vi "LED logic.vi"(11 "Blinks per cycle":i32) -> (3 "Boolean":bool)   [LabVIEW 2013, in "LED runtime.lvclass"]
uses:
  LED runtime.lvclass
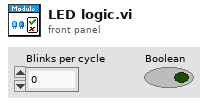
[diagram p1: front panel]
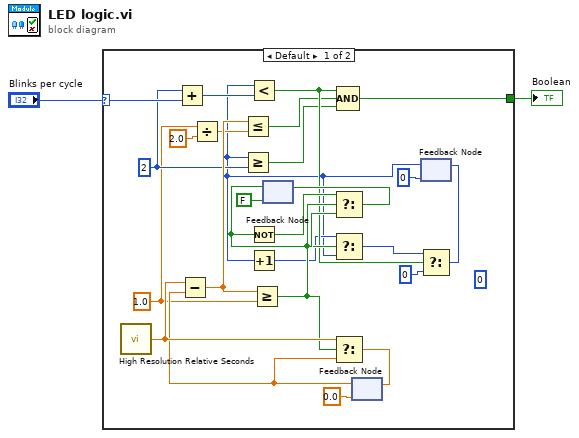
[diagram p0: block diagram]
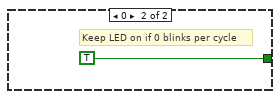
[diagram p2: hidden frame]
diagram:
  n1 = case shown="Default" "Blinks per cycle" {
    selector: "Blinks per cycle" -> [w9 _]
    tunnel: [w12 TRUE] -> w1
    frame Default {
      w3 = 1.0
      (unwired) 0 ("f")
      w7 = 2 ("x")
      n2 = call <vilib>:"High Resolution Relative Seconds.vi"() -> ("relative seconds"=w23:dbl)
      n3 = Add(x=w7, y=w9) -> (x+y=w8:i32)
      n4 = Divide(x=w3, y=2.0) -> (x/y=w13:dbl)
      n5 = feedback #1(FALSE) -> (w24:bool)
      n6 = Not(x=w24) -> (.not. x?=w26:bool)
      n7 = feedback #2(0.0) -> (w22:dbl)
      n8 = Subtract(x=w23, y=w22) -> (x-y=w15:dbl)
      n9 = Less Or Equal?(x=w15, y=w13) -> (x <= y?=w10:bool)
      n10 = Greater Or Equal?(x=w15, y=w3) -> (x >= y?=w17:bool)
      n11 = Select(t=w26, s=w17, f=w24) -> (s? t:f=w25:bool)
      n12 = feedback-in #1(w25) -> ()
      n13 = Select(t=w23, s=w17, f=w22) -> (s? t:f=w21:dbl)
      n14 = feedback-in #2(w21) -> ()
      n15 = feedback #3(0 ("Blinks per cycle")) -> (w4:i32)
      n16 = Greater Or Equal?(x=w4, y=w7) -> (x >= y?=w6:bool)
      n17 = Less?(x=w4, y=w8) -> (x < y?=w11:bool)
      n18 = Increment(x=w4) -> (x+1=w5:i32)
      n19 = Select(t=w5, s=w17, f=w4) -> (s? t:f=w16:i32)
      n20 = Compound Arithmetic op=AND(w11, w10, w6) -> (w12:bool)
      n21 = Select(t=w16, s=w11, f=0) -> (s? t:f=w18:i32)
      n22 = feedback-in #3(w18) -> ()
    }
    frame 0 {
      # "Keep LED on if 0 blinks per cycle"
    }
  }
  "Boolean" <- w1
